vi "Gamma PID - V2.vi"(6 "nonzero temperature":dbl=300.0, 10 "sweep folder path":path, 11 "adaptive parameters":T1={"peaks are known -- parameters"={"Def Gamma (kHz)"=0.5, "dV"=17.0, "time in Gamma (sec)"=7.0, "phi-star"=0.0, "all peaks (kHz)"=[], "delta t (sec)"=22.0, "default step (Hz)"=0.0, "all gamma (kHz)"=[564.0, 649.0, 987.0, 1133.0, 1214.0, 1585.0, 1763.0, 1823.0, 1880.0, 1899.0, 2032.0, 2138.0, 2221.0, 2270.0, 2350.0, 2456.0, 2580.0, 2634.0, 2831.0, 2960.0, 2965.0, 3131.0, 3328.0, 3469.0, 3553.0, 0.0, 3615.0, 3734.0, 0.0, 0.0, 0.0, 4236.0, 4300.0, 4331.0], "peaks OK"=FALSE, "gamma OK"=FALSE, "near omega (kHz)"=0.0, "near gamma (kHz)"=0.0, "min step (Hz)"=10000.0, "max step(Hz)"=0.01, "min gamma (kHz)"=0.01, "all time in gamma (sec)"=[], "time in gamma OK"=FALSE, "time-in-gamma mode"=enum."same for all"}, "find peak - parameters"={"wavepacket"={"R"=0.5, "wave number"=17.0, "delta k"=7.0, "radii vector"=[], "radial section"=[], "wave vector"=22.0, "wavepacket is"=TRUE}, "number of grid points"=70, "decimation threshold"=1, "Voltage range"=0.1, "target freq step"=20.0, "target spot size"=0.05, "factor"=1.0, "another factor"=1.0, "analyze last # sec"=3, "scale factor"=3}} {"find peak - parameters"."wavepacket"."delta k" format="%#_3f"; "find peak - parameters"."wavepacket"."wave number" format="%#_3f"; "find peak - parameters"."wavepacket"."R" format="%#_3f"}) -> (0 "Peaks OK":bool, 3 "adaptive parameters out":T1={"peaks are known -- parameters"={"Def Gamma (kHz)"=0.5, "dV"=17.0, "time in Gamma (sec)"=7.0, "phi-star"=0.0, "all peaks (kHz)"=[], "delta t (sec)"=22.0, "default step (Hz)"=0.0, "all gamma (kHz)"=[564.0, 649.0, 987.0, 1133.0, 1214.0, 1585.0, 1763.0, 1823.0, 1880.0, 1899.0, 2032.0, 2138.0, 2221.0, 2270.0, 2350.0, 2456.0, 2580.0, 2634.0, 2831.0, 2960.0, 2965.0, 3131.0, 3328.0, 3469.0, 3553.0, 0.0, 3615.0, 3734.0, 0.0, 0.0, 0.0, 4236.0, 4300.0, 4331.0], "peaks OK"=FALSE, "gamma OK"=FALSE, "near omega (kHz)"=0.0, "near gamma (kHz)"=0.0, "min step (Hz)"=10000.0, "max step(Hz)"=0.01, "min gamma (kHz)"=0.01, "all time in gamma (sec)"=[], "time in gamma OK"=FALSE, "time-in-gamma mode"=enum."same for all"}, "find peak - parameters"={"wavepacket"={"R"=0.5, "wave number"=17.0, "delta k"=7.0, "radii vector"=[], "radial section"=[], "wave vector"=22.0, "wavepacket is"=TRUE}, "number of grid points"=70, "decimation threshold"=1, "Voltage range"=0.1, "target freq step"=20.0, "target spot size"=0.05, "factor"=1.0, "another factor"=1.0, "analyze last # sec"=3, "scale factor"=3}} {"find peak - parameters"."wavepacket"."delta k" format="%#_3f"; "find peak - parameters"."wavepacket"."wave number" format="%#_3f"; "find peak - parameters"."wavepacket"."R" format="%#_3f"})   [LabVIEW 2015]
uses:
  single sweep - adaptive parameters.ctl
  next chunk -- parameters.ctl
  time in gamma mode control.ctl
  find peak -- parameters.ctl
  wavepacket.ctl
  ctl -- name dispatcher -- action.ctl
  next chunk - read-write freq PID file - atomic actions .vi
  ctl -- name dispatcher.vi
  file -- 9w path.vi
  array -- find index - real.vi
  array -- interpolate -- i.vi
  Q -- check range -- i -- real.vi
  Q - not nan -- real.vi
  <vilib>/Utility/libraryn.llb/Check if File or Folder Exists.vi
  file -- read list of lines.vi
  parse -- find first line.vi
  parse -- get list of matches -- numbers.vi
  <vilib>/Utility/file.llb/Write To Spreadsheet File.vi
  <vilib>/Utility/file.llb/Write To Spreadsheet File (string).vi
  <vilib>/gmath/function.llb/Binomial Coefficient.vi
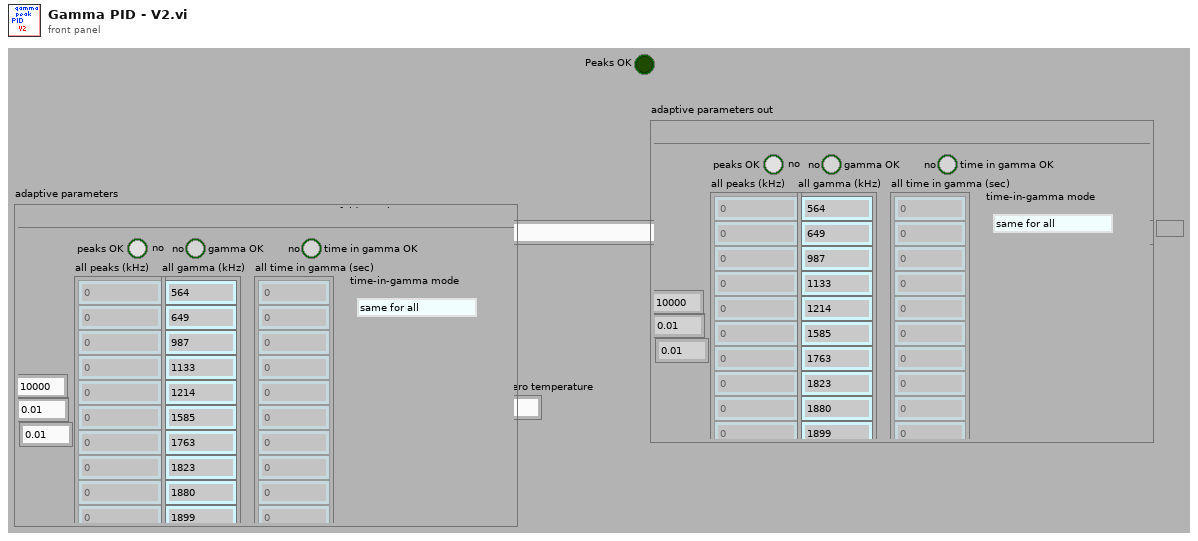
[diagram p1: front panel]
types:
  T1 = typedef "single sweep - adaptive parameters.ctl" = cluster{"peaks are known -- parameters":T2, "find peak - parameters":T4}
  T2 = typedef "next chunk -- parameters.ctl" = cluster{"Def Gamma (kHz)":dbl, "dV":dbl, "time in Gamma (sec)":dbl, "phi-star":dbl, "all peaks (kHz)":dbl[], "delta t (sec)":dbl, "default step (Hz)":dbl, "all gamma (kHz)":dbl[], "peaks OK":bool, "gamma OK":bool, "near omega (kHz)":dbl, "near gamma (kHz)":dbl, "min step (Hz)":dbl, "max step(Hz)":dbl, "min gamma (kHz)":dbl, "all time in gamma (sec)":dbl[], "time in gamma OK":bool, "time-in-gamma mode":T3}
  T3 = typedef "time in gamma mode control.ctl" = enum16{"same for all", "each one different", "uniform scan"}
  T4 = typedef "find peak -- parameters.ctl" = cluster{"wavepacket":T5, "number of grid points":i32, "decimation threshold":i32, "Voltage range":dbl, "target freq step":dbl, "target spot size":dbl, "factor":dbl, "another factor":dbl, "analyze last # sec":i32, "scale factor":i32}
  T5 = typedef "wavepacket.ctl" = cluster{"R":dbl, "wave number":dbl, "delta k":dbl, "radii vector":dbl[], "radial section":cdb[], "wave vector":dbl, "wavepacket is":bool}
  T6 = typedef "ctl -- name dispatcher -- action.ctl" = enum16{"peak frequency", "peak frequency DUMP", "peak gamma DUMP", "peak gamma", "peak frequency TEST", "peak gamma TEST", "ultrasonic power", "time in gamma", "set temperature ", "set temperature timer", "peak default gamma", "last scan file", "peak freq gamma TEST", "peak NAMES", "errors", "P_I_D", "P", "I", "D", "power vs time", "power vs time TIMER", "void", "power log", "set temperature - SINE", "itc ltc log", "peak - time in gamma"}
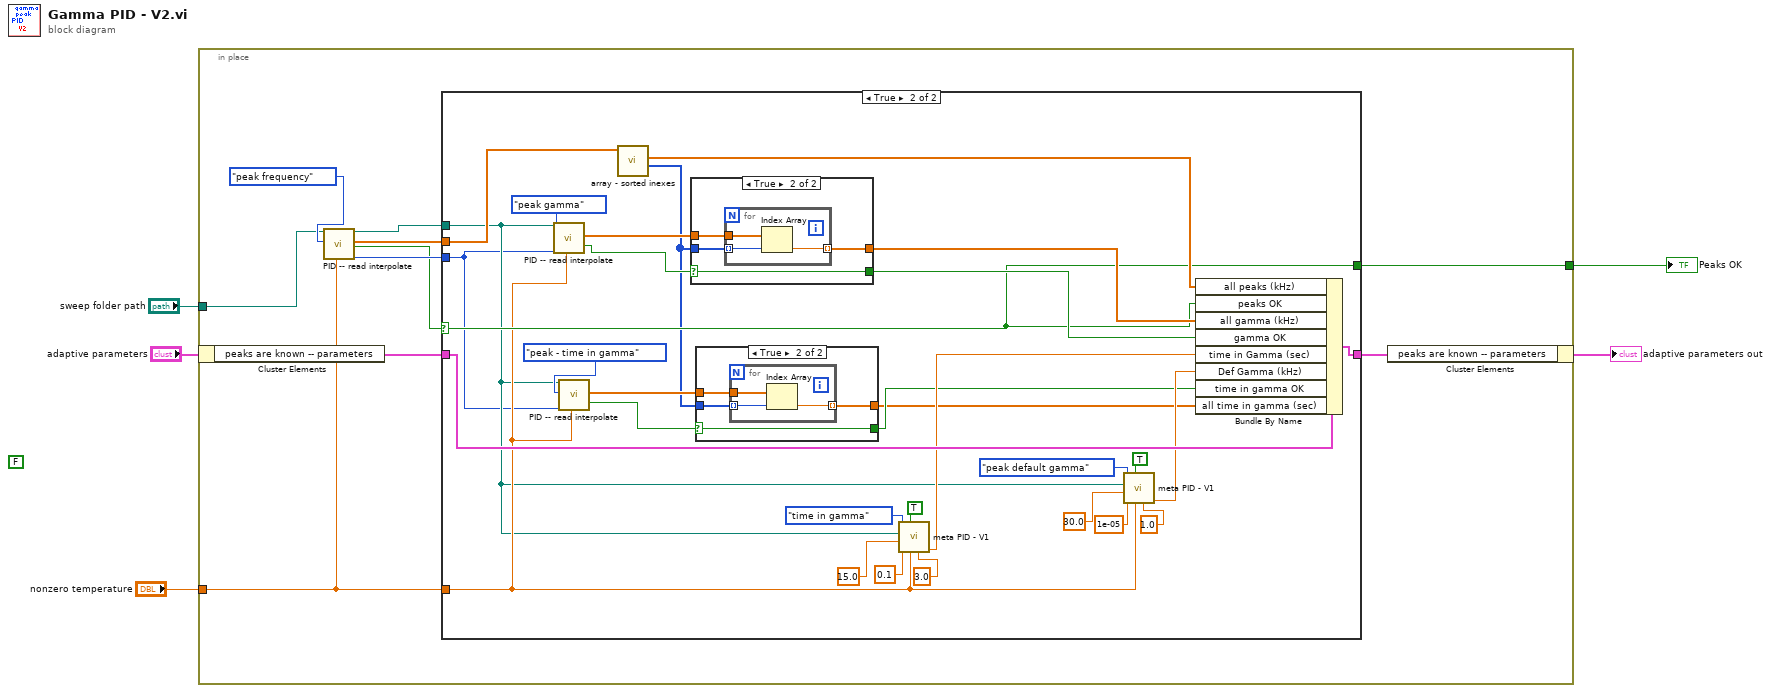
[diagram p0: block diagram]
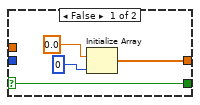
[diagram p3: hidden frame]
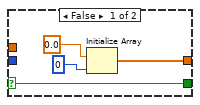
[diagram p4: hidden frame]
diagram:
  (unwired) FALSE ("peaks are known -- parameters.peaks OK")
  n1 = in-place {
    in-place-border: "sweep folder path" -> [w11]
    in-place-border: "nonzero temperature" -> [w10]
    in-place-border: [w6] -> w1
    n2 = in-place-cluster #1("adaptive parameters") -> ("peaks are known -- parameters"=w8:T2)
    n3 = call "PID -- read interpolate.vi"("sweep folder path"=w11, "ctl PID file IN"=ctl_--_name_dispatcher_--_action."peak frequency", "temperature"=w10) -> ("sweep folder path out"=w14:path, "PID freq"=w12:dbl[], "PID OK !"=w9:bool, "length out"=w13:i32)  [unwired: 11 in, 2 out]
    n4 = case shown="True" w9 {
      selector: w9 -> [w16 w32]
      tunnel: w14 -> [_ w24]
      tunnel: w13 -> [_ w22]
      tunnel: w12 -> [_ w43]
      tunnel: w10 -> [_ w25]
      tunnel: w8 -> [w17 w42]
      tunnel: [w17 w33] -> w7
      tunnel: [w16 w32] -> w6
      frame False {
      }
      frame True {
        n5 = call "PID -- read interpolate.vi"("sweep folder path"=w24, "ctl PID file IN"=ctl_--_name_dispatcher_--_action."peak gamma", "length"=w22, "temperature"=w25) -> ("PID freq"=w39:dbl[], "Length OK !"=w23:bool)  [unwired: 10 in, 4 out]
        n6 = call "PID -- read interpolate.vi"("sweep folder path"=w24, "ctl PID file IN"=ctl_--_name_dispatcher_--_action."peak - time in gamma", "length"=w22, "temperature"=w25) -> ("PID freq"=w26:dbl[], "Length OK !"=w21:bool)  [unwired: 10 in, 4 out]
        n7 = call "array - sorted inexes.vi"("x"=w43) -> ("index array"=w18:i32[], "sorted array"=w41:dbl[])  [unwired: 9 in]
        n8 = case shown="True" w23 {
          selector: w23 -> [w62 w67]
          tunnel: [w62 w67] -> w40
          tunnel: w39 -> [_ w66]
          tunnel: w18 -> [_ w65]
          tunnel: [w61 w64] -> w38
          frame False {
            n9 = Initialize Array(0.0 ("index"), 0 ("index")) -> (w61:dbl[])
          }
          frame True {
            n10 = for {
              tunnel: w66 -> [w70]
              tunnel: w65 -> [w69] mode=indexing
              tunnel: [w68] -> w64 mode=indexing
              n11 = Index Array(array=w70, index=w69) -> (element=w68:dbl)
            }
          }
        }
        n12 = case shown="True" w21 {
          selector: w21 -> [w51 w56]
          tunnel: [w51 w56] -> w20
          tunnel: w26 -> [_ w55]
          tunnel: [w50 w54] -> w19
          tunnel: w18 -> [_ w53]
          frame False {
            n13 = Initialize Array(0.0 ("index"), 0 ("index")) -> (w50:dbl[])
          }
          frame True {
            n14 = for {
              tunnel: w55 -> [w59]
              tunnel: [w58] -> w54 mode=indexing
              tunnel: w53 -> [w57] mode=indexing
              n15 = Index Array(array=w59, index=w57) -> (element=w58:dbl)
            }
          }
        }
        n16 = call "meta PID - V1.vi"("default output"=3.0 ("lower"), "input parameter"=w25, "control?"=TRUE ("control power PID?"), "lower limit"=0.1 ("lower"), "upper limit"=15.0 ("upper"), "sweep folder path"=w24, "ctl name dispatch"=ctl_--_name_dispatcher_--_action."time in gamma") -> ("bezier output"=w30:dbl)  [unwired: 1 in, 3 out]
        n17 = call "meta PID - V1.vi"("default output"=1.0 ("lower"), "input parameter"=w25, "control?"=TRUE ("control power PID?"), "lower limit"=1e-05 ("lower"), "upper limit"=30.0 ("upper"), "sweep folder path"=w24, "ctl name dispatch"=ctl_--_name_dispatcher_--_action."peak default gamma") -> ("bezier output"=w28:dbl)  [unwired: 1 in, 3 out]
        n18 = Bundle By Name(cluster=w42, "all peaks (kHz)"=w41, "peaks OK"=w32, "all gamma (kHz)"=w38, "gamma OK"=w40, "time in Gamma (sec)"=w30, "Def Gamma (kHz)"=w28, "time in gamma OK"=w20, "all time in gamma (sec)"=w19) -> (w33:T2)
      }
    }
    n19 = in-place-cluster #1("peaks are known -- parameters"=w7) -> (→"adaptive parameters out":T1)
  }
  "Peaks OK" <- w1
